vi "Get DataRef Create SV.vi"(11 "Device Ref in":T2=18446744073709551615 format="%.0x") -> (0 "Ausgangs-Cluster":T1 {"Channel Data Reference" format="%.0x"; "Dep. Channel Refs" format="%.0x"})   [LabVIEW 2013, in "Datadashboard CD Custom Device.lvlib"]
uses:
  Datadashboard CD Custom Device.lvlib
  <vilib>/NI Veristand/Custom Device API/Custom Device Item Ref.ctl
  Channel Block Ref.ctl
  <vilib>/NI Veristand/Custom Device API/Data Reference.ctl
  <vilib>/NI Veristand/Custom Device API/Custom Device API.lvlib
  <vilib>/NI Veristand/Custom Device Tools/Custom Device Utility Library/Custom Device Utility Library.lvlib
  <vilib>/lvdsc/NI_DSC.lvlib
panel:
  in  "Channel Block Ref":T1 {"Channel Data Reference" format="%.0x"; "Dep. Channel Refs" format="%.0x"}
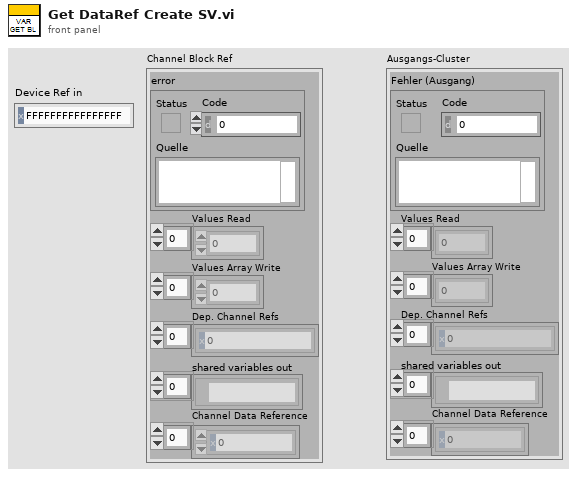
[diagram p1: front panel]
types:
  T1 = typedef "Channel Block Ref.ctl" = cluster{"error":errorcluster, "Values Read":dbl[], "Values Array Write":dbl[], "Dep. Channel Refs":T2[], "shared variables out":refnum<k21>[], "Channel Data Reference":T3[]}
  T2 = typedef "Custom Device API.lvlib/Custom Device Item Ref.ctl" = u64
  T3 = typedef "Custom Device API.lvlib/Data Reference.ctl" = i32
  T4 = enum32{"u32BitField", "bool", "double", "string", "int8", "uint8", "int16", "uint16", "int32", "uint32", "int64", "uint64", "single", "double waveform", "int16 waveform", "array of boolean", "array of int8", "array of uint8", "array of int16", "array of uint16", "array of int32", "array of uint32", "array of int64", "array of uint64", "array of single", "array of double", "array of double waveform", "array of int16 waveform", "array of string", "variant", "timestamp", "fixed point", "custom"}
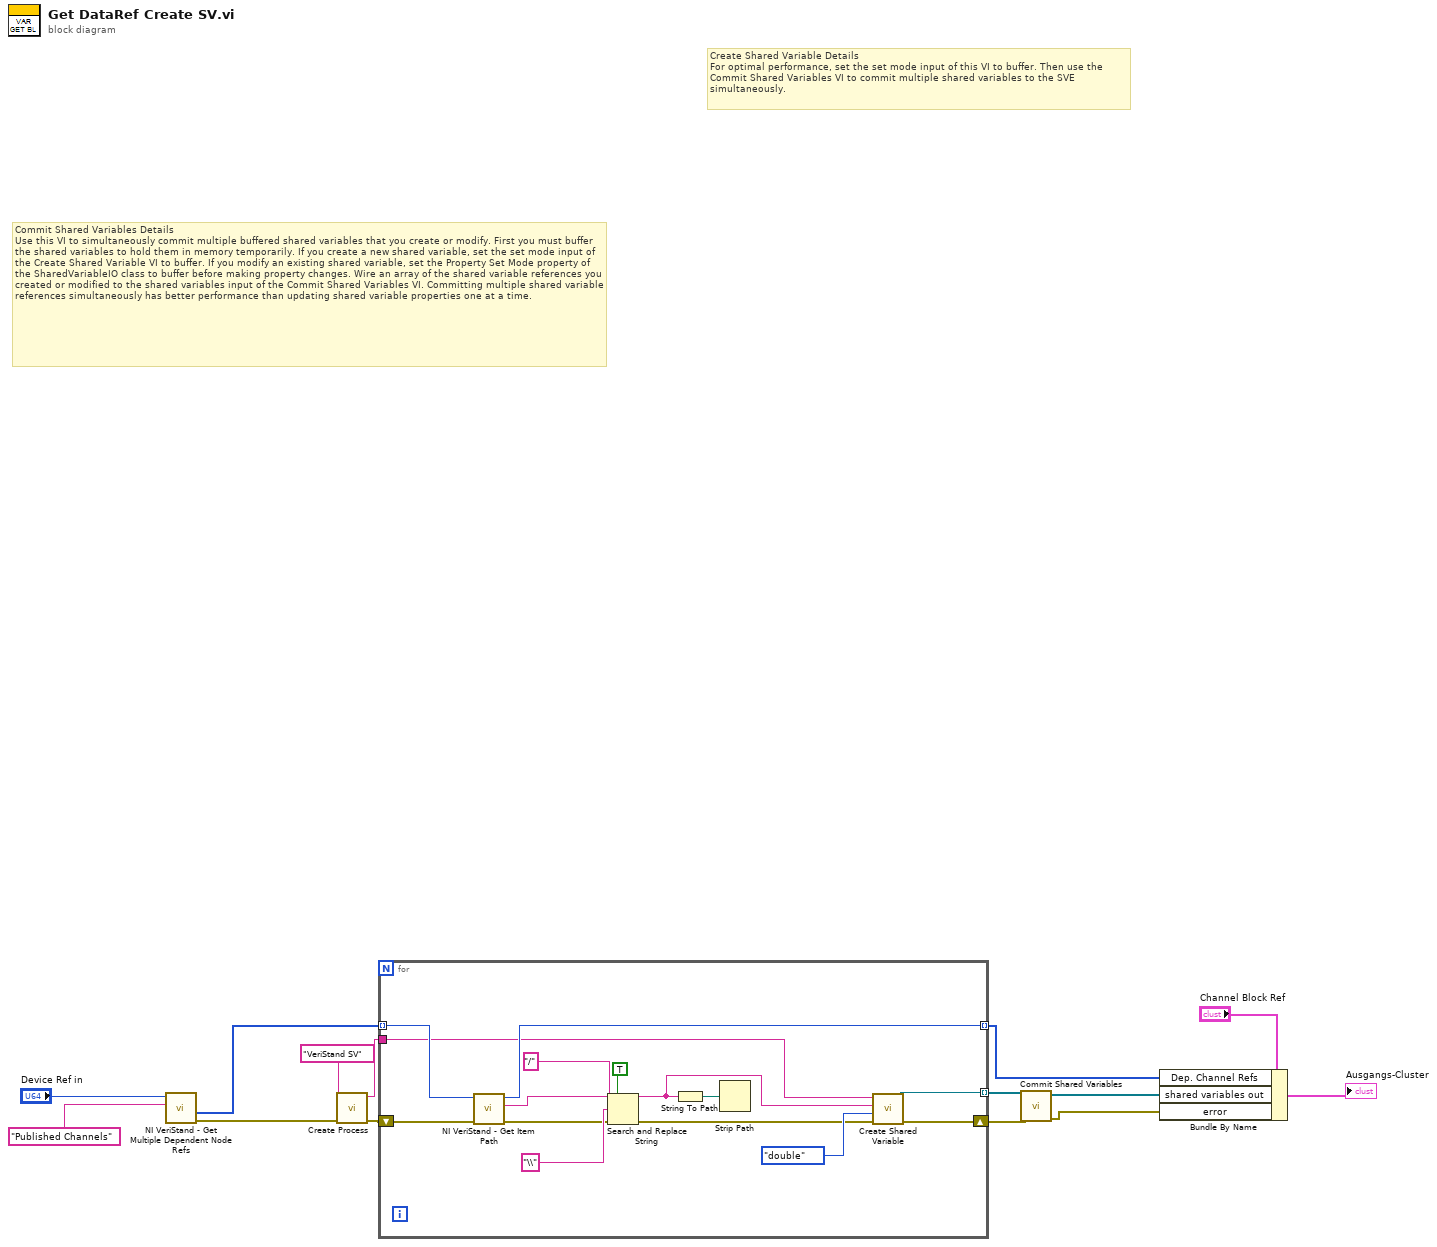
[diagram p0: block diagram]
diagram:
  # "Commit Shared Variables Details\nUse this VI to simultaneously commit multiple buffered shared variables that you create or modify. First you must buffer the shared variables to hold them in memory temporarily. If you create a new shared variable, set the set mode input of the Create Shared Variable VI to buffer. If you modify an existing shared variable, set the Property Set Mode property of the SharedVariableIO class to buffer before making property changes. Wire an array of the shared variable references you created or modified to the shared variables input of the Commit Shared Variables VI. Committing multiple shared variable references simultaneously has better performance than updating shared variable properties one at a time."
  # "Create Shared Variable Details\nFor optimal performance, set the set mode input of this VI to buffer. Then use the Commit Shared Variables VI to commit multiple shared variables to the SVE simultaneously."
  n1 = call <vilib>:"NI VeriStand - Get Multiple Dependent Node Refs.vi"("Base Property Name"="Published Channels" ("Property Name"), "Item Ref in"="Device Ref in") -> ("error out"=w6:errorcluster, "Dependent Node Refs"=w10:T2[])  [unwired: 7 in, 1 out]
  n2 = call <vilib>:"Create Process.vi"("error in (no error)"=w6, "process name"="VeriStand SV") -> ("error out"=w5:errorcluster, "process name out"=w4:string)  [unwired: 8 in]
  n3 = for {
    shift-right: [w25] -> w3
    shift-left: w5 -> [w27]
    tunnel: w10 -> [w28] mode=indexing
    tunnel: [w26] -> w9 mode=indexing
    tunnel: w4 -> [w24]
    tunnel: [w29] -> w1 mode=indexing
    n4 = call <vilib>:"NI VeriStand - Get Item Path.vi"("error in (no error)"=w27, "Item Ref in"=w28) -> ("error out"=w16:errorcluster, "Path"=w23:string, "Item Ref out"=w29:T2)  [unwired: 6 in, 1 out]
    n5 = Search and Replace String(replace all?=TRUE ("Alle ersetzen? (F)"), input string=w23, search string="/" ("Such-String"), replace string="\\" ("String ersetzen(\"\")"), error in=w16) -> (result string=w17:string, error out=w15:errorcluster)  [unwired: 3 in, 2 out]
    n6 = String To Path(string=w17) -> (path=w21:path)
    n7 = Strip Path(path=w21) -> ()  [unwired: 2 out]
    n8 = call <vilib>:"Create Shared Variable.vi"("error in (no error)"=w15, "data type"=T4."double", "shared variable name"=w17, "process name"=w24) -> ("error out"=w25:errorcluster, "shared variable"=w26:refnum<k21>)  [unwired: 5 in, 1 out]
  }
  n9 = call <vilib>:"Commit Shared Variables.vi"("error in (no error)"=w3, "shared variables"=w9) -> ("error out"=w2:errorcluster, "shared variables out"=w8:refnum<k21>[])  [unwired: 8 in]
  n10 = Bundle By Name(cluster="Channel Block Ref", "Dep. Channel Refs"=w1, "shared variables out"=w8, "error"=w2) -> (→"Ausgangs-Cluster":T1)
